vi "cmd.vi"() -> ()   [LabVIEW 2020]
doc: "This examples launches the cmd.exe process and allows you to send strings via stdin, while asynchronously listening to stdout and stderr \n\nCalling \"exit\" in CmdIn will stop the cmd.exe instance and stop this VI. You can leverage this by adding a final exit line after the command(s)\nyou wish to send to have this VI auto-terminate upon completion.\n\n-----------------------------------------------\nJKI .NET System Exec 1.0.0.6\nJavier Ruiz - JKI\nCopyright (c) 2021, JKI\njki.net"
uses:
  Instrument/Typedefs/Data.ctl
  Instrument/Instrument.lvclass
  C:/Program Files (x86)/National Instruments/LabVIEW 2020/vi.lib/JKI/JKI SMO/SMO/SMO.lvclass
  <vilib>/JKI/JKI DotNet System Exec/dotnet_system_exec/dotnet_system_exec.lvclass
  <vilib>/JKI/JKI SMO/SMO/SMO.lvclass
panel:
  out "new instrument data":T1
  in  "Send to UI":bool
  in  "Data":string
  in  "Shutdown":bool
  in  "working directory":path=path "C:/Data/dump1090-win.1.10.3010.14"
  out "StdErr":string
  out "StdOut":string
  in  "Send":bool
  in  "Cmd In (can include multiple lines)":string="dump1090.exe --interactive --net --net-beast --net-http-port 8081"
  in  "Stop":bool
  # "This examples launches the cmd.exe process and allows you to send strings via stdin, while asynchronously listening to stdout and stderr  \n\nCalling \"exit\" in CmdIn will stop the cmd.exe instance and stop this VI. You can leverage this by adding a final exit line after the command(s)\nyou wish to send to have this VI auto-terminate upon completion."
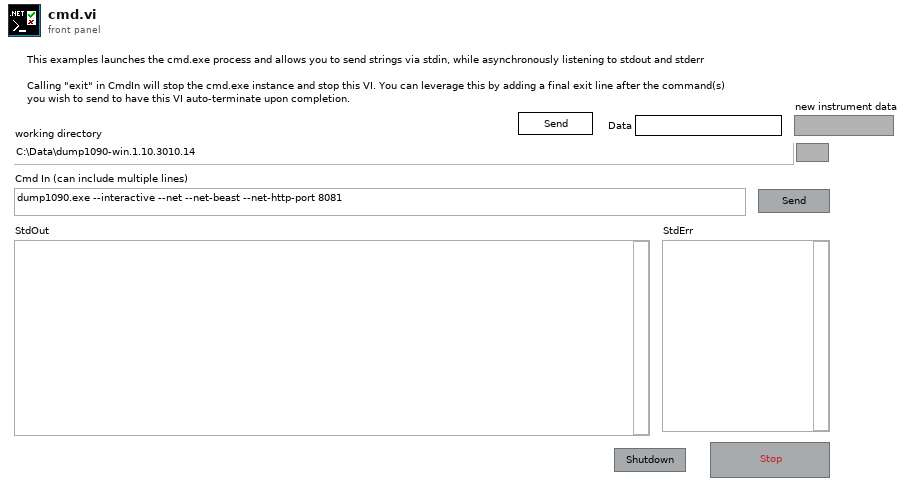
[diagram p1: front panel]
types:
  T1 = typedef "Instrument.lvclass/Data.ctl" = string
  T2 = typedef "Instrument.lvclass/PublicEvents--Cluster.ctl" = cluster{"Data Changed":refnum<user-event>}
  T3 = cluster{"stdout event":refnum<user-event>, "stderr event":refnum<user-event>, "process_exit event":refnum<user-event>}
  T4 = typedef "SMO.lvclass/Public Events.ctl" = cluster{"Error":refnum<user-event>, "State":refnum<user-event>, "Reserve State":refnum<user-event>}
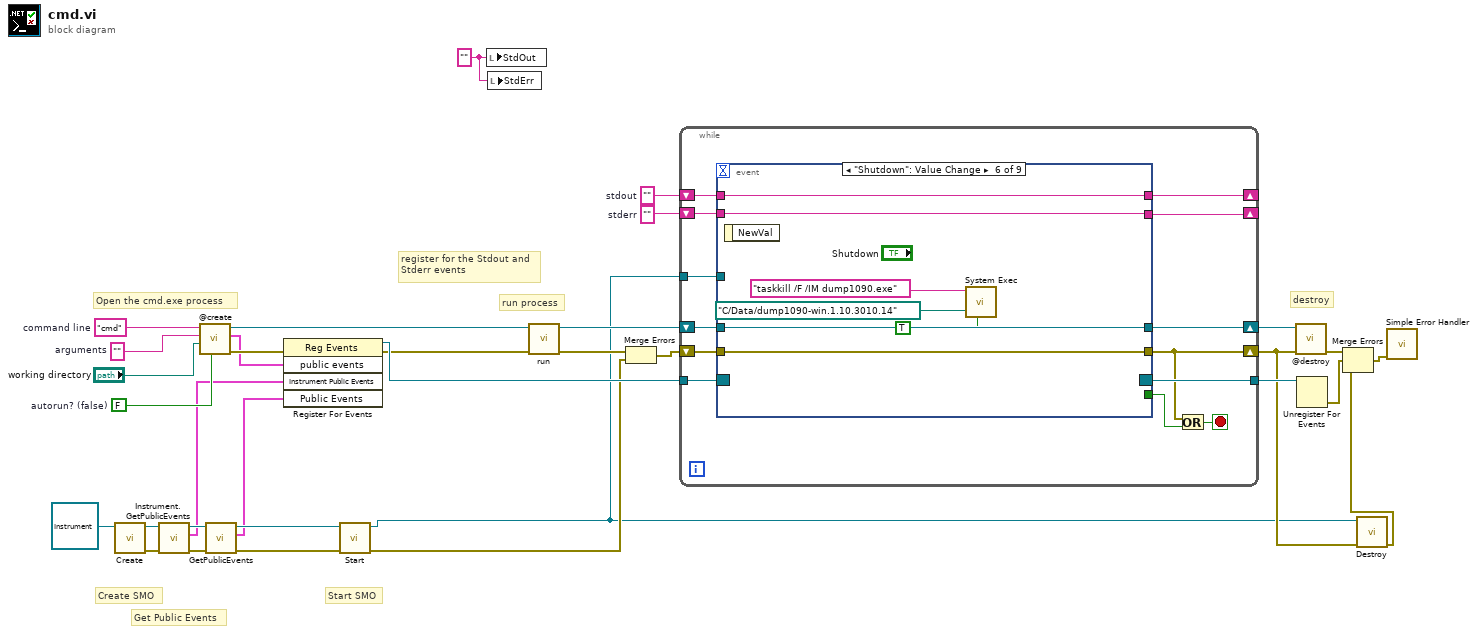
[diagram p0: block diagram]
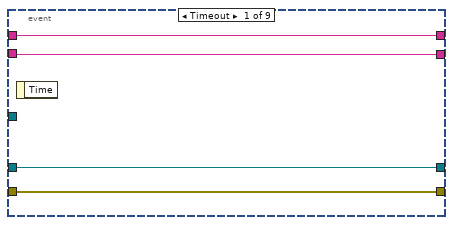
[diagram p2: hidden frame]
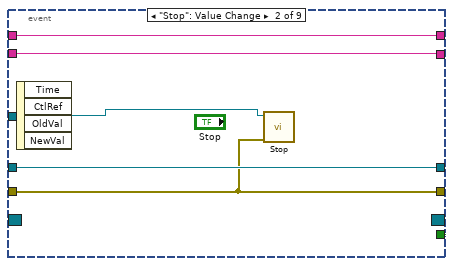
[diagram p3: hidden frame]
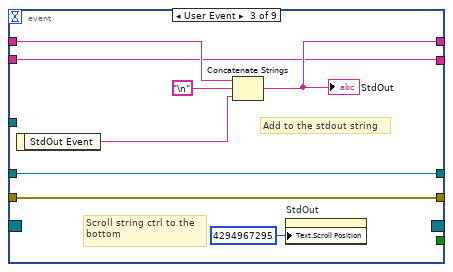
[diagram p4: hidden frame]
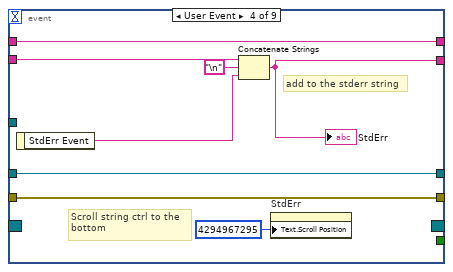
[diagram p5: hidden frame]
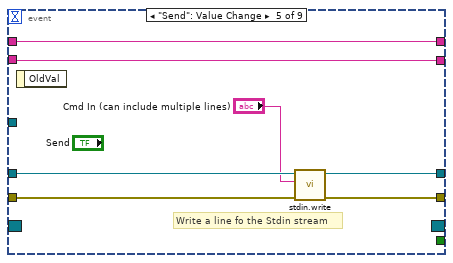
[diagram p6: hidden frame]
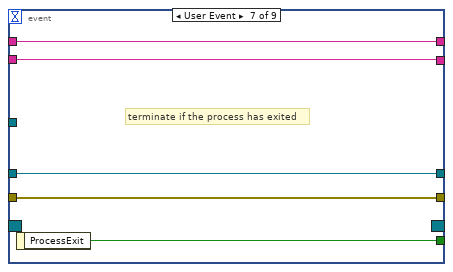
[diagram p7: hidden frame]
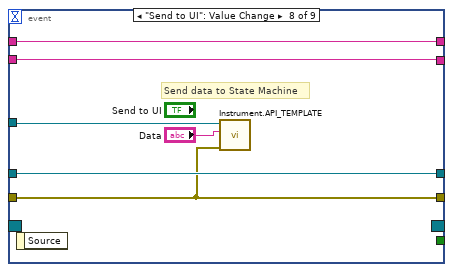
[diagram p8: hidden frame]
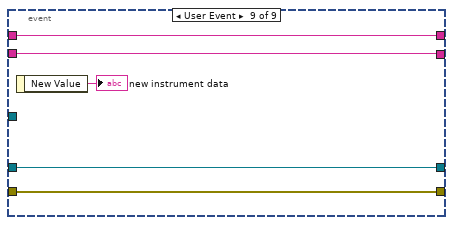
[diagram p9: hidden frame]
diagram:
  w16 = FALSE  # autorun? (false)
  w17 = "" ("Process File Name")
  w19 = ""  # stderr
  w24 = ""  # arguments
  w25 = ""  # stdout
  w26 = "cmd"  # command line
  # "Get Public Events"
  # "Start SMO"
  # "Create SMO"
  # "destroy"
  # "register for the Stdout and\nStderr events"
  # "run process"
  # "Open the cmd.exe process"
  n1 = call <vilib>:"Create.vi"("SMO"=refnum<class "Instrument.lvclass"> refnum ("SMO.Template.lvclass")) -> ("error out"=w13:errorcluster, "SMO out"=w14:refnum<class "Instrument.lvclass">)  [unwired: 8 in, 1 out]
  n2 = call "Instrument.GetPublicEvents.vi"("error in (no error)"=w13, "Instrument"=w14) -> ("error out"=w10:errorcluster, "Instrument Public Events"=w8:T2, "Instrument out"=w12:refnum<class "Instrument.lvclass">)  [unwired: 7 in]
  n3 = call <vilib>:"@create.vi"("autorun? (false)"=w16, "working directory (c:\\)"="working directory", "arguments (\"\")"=w24, "command line (cmd.exe)"=w26) -> ("error out"=w22:errorcluster, "public events"=w20:T3, "dotnet_system_exec out"=w31:refnum<class "dotnet_system_exec.lvclass">)  [unwired: 5 in]
  n4 = call <vilib>:"GetPublicEvents.vi"("error in (no error)"=w10, "SMO"=w12) -> ("error out"=w9:errorcluster, "Public Events"=w7:T4, "SMO out"=w11:refnum<class "Instrument.lvclass">)  [unwired: 7 in]
  n5 = register-events(error in=w22, w20, w8, w7) -> (reference out=w30:refnum<event-registration>, error out=w21:errorcluster)  [unwired: 1 in]
  n6 = call <vilib>:"Start.vi"("error in (no error)"=w9, "SMO"=w11) -> ("error out"=w3:errorcluster, "SMO out"=w1:refnum<class "Instrument.lvclass">)  [unwired: 8 in]
  n7 = local write "StdOut"(w17) -> ()
  n8 = local write "StdErr"(w17) -> ()
  n9 = call <vilib>:"run.vi"("error in (no error)"=w21, "dotnet_system_exec in"=w31) -> ("error out"=w23:errorcluster, "dotnet_system_exec out"=w33:refnum<class "dotnet_system_exec.lvclass">)  [unwired: 8 in]
  n10 = Merge Errors(w23, w3) -> (w4:errorcluster)
  n11 = while {
    shift-right: [w46] -> w32
    shift-left: w33 -> [w45]
    shift-right: [w36] -> w5
    shift-left: w4 -> [w44]
    tunnel: w30 -> [w43]
    tunnel: [w42] -> w29
    shift-right: [w40] -> _
    shift-left: w25 -> [w41]
    shift-right: [w38] -> _
    shift-left: w19 -> [w39]
    tunnel: w1 -> [w34]
    stop <- w35 stop-if-true
    n12 = event shown="[5] \"Shutdown\": Value Change" {
      selector: w43 -> [_ _ _ _ _ _ _ _ _]
      dyn-events: [_ _ _ _ _ _ _ _ _] -> w42
      timeout: _ -> [_ _ _ _ _ _ _ _ _]
      tunnel: [w50 w56 w64 w72 w79 w86 w88 w97 w102] -> w46
      tunnel: w45 -> [w50 w56 w64 w72 w78 w86 w88 w97 w102]
      tunnel: w44 -> [w49 w52 w63 w71 w76 w85 w87 w92 w101]
      tunnel: [w49 w52 w63 w71 w77 w85 w87 w92 w101] -> w36
      tunnel: w41 -> [w48 w54 w60 w67 w74 w84 w89 w96 w100]
      tunnel: [w48 w54 w61 w67 w74 w84 w89 w96 w100] -> w40
      tunnel: [_ TRUE _ _ _ _ w91 _ _] -> w37
      tunnel: w39 -> [w47 w53 w58 w68 w73 w83 w90 w95 w99]
      tunnel: [w47 w53 w58 w66 w73 w83 w90 w95 w99] -> w38
      tunnel: w34 -> [_ w51 _ _ _ _ _ w93 _]
      event Timeout {
        n13 = event-data() -> ()  [unwired: 1 in, 1 out]
      }
      event "Stop": Value Change {
        n14 = event-data() -> ()  [unwired: 1 in, 4 out]
        n15 = call <vilib>:"Stop.vi"("error in (no error)"=w52, "SMO"=w51) -> ()  [unwired: 8 in, 2 out]
      }
      event User Event {
        # "Scroll string ctrl to the \nbottom"
        # "Add to the stdout string"
        n16 = event-data() -> ("StdOut Event"=w59:string)  [unwired: 1 in]
        n17 = Concatenate Strings(w60, "\n", w59) -> (w61:string)
        "StdOut" <- w61
        n18 = property on="StdOut" class="Str"("Text.Scroll Position"=u32 4294967295) -> ()  [unwired: 2 in, 2 out]
      }
      event User Event {
        # "Scroll string ctrl to the \nbottom"
        # "add to the stderr string"
        n19 = event-data() -> ("StdErr Event"=w69:string)  [unwired: 1 in]
        n20 = Concatenate Strings(w68, "\n", w69) -> (w66:string)
        "StdErr" <- w66
        n21 = property on="StdErr" class="Str"("Text.Scroll Position"=u32 4294967295) -> ()  [unwired: 2 in, 2 out]
      }
      event "Send": Value Change {
        # "Write a line fo the Stdin stream"
        n22 = event-data() -> ()  [unwired: 1 in, 1 out]
        n23 = call-dynamic "stdin.write.vi"("error in (no error)"=w76, "stdin"="Cmd In (can include multiple lines)", "dotnet_system_exec in"=w78) -> ("error out"=w77:errorcluster, "dotnet_system_exec out"=w79:refnum<class "dotnet_system_exec.lvclass">)  [unwired: 7 in]
      }
      event "Shutdown": Value Change {
        n24 = event-data() -> ()  [unwired: 1 in, 1 out]
        n25 = call <vilib>:"System Exec.vi"("run minimized? (F)"=TRUE, "working directory"=path "C:/Data/dump1090-win.1.10.3010.14", "command line"="taskkill /F /IM dump1090.exe") -> ()  [unwired: 5 in, 4 out]
      }
      event User Event {
        # "terminate if the process has exited"
        n26 = event-data() -> ("ProcessExit"=w91:bool)  [unwired: 1 in]
      }
      event "Send to UI": Value Change {
        # "Send data to State Machine"
        n27 = event-data() -> ()  [unwired: 1 in, 1 out]
        n28 = call "Instrument.API_TEMPLATE.vi"("error in (no error)"=w92, "Data"="Data", "Instrument"=w93) -> ()  [unwired: 7 in, 2 out]
      }
      event User Event {
        n29 = event-data() -> ("New Value"=→"new instrument data":T1)  [unwired: 1 in]
      }
    }
    n30 = Or(x=w36, y=w37) -> (x .or. y?=w35:bool)
  }
  n31 = call-dynamic "@destroy.vi"("error in (no error)"=w5, "dotnet_system_exec in"=w32) -> ("error out"=w28:errorcluster)  [unwired: 8 in, 1 out]
  n32 = Unregister For Events(event registration refnum=w29) -> (error out=w6:errorcluster)  [unwired: 1 in]
  n33 = call <vilib>:"Destroy.vi"("error in (no error)"=w5, "SMO"=w1) -> ("error out"=w2:errorcluster)  [unwired: 9 in]
  n34 = Merge Errors(w28, w6, w2) -> (w27:errorcluster)
  n35 = call <vilib>:"Simple Error Handler.vi"("error in (no error)"=w27) -> ()  [unwired: 4 in, 5 out]
